vi "UTIL Config Analog Output_v3.vi"(0 "physical channels":tag) -> (1 "sampling info":cluster{"Fs":dbl, "#s":dbl}, 2 "error out":errorcluster, 3 "task out":refnum<k21>)   [LabVIEW 2010]
uses:
  <vilib>/DAQmx/create/channels.llb/DAQmx Create Channel (AO-Voltage-Basic).vi
  <vilib>/DAQmx/configure/timing.llb/DAQmx Timing (Sample Clock).vi
  Program Files (x86)/National Instruments/LabVIEW 2010/resource/objmgr/daqmx.rc
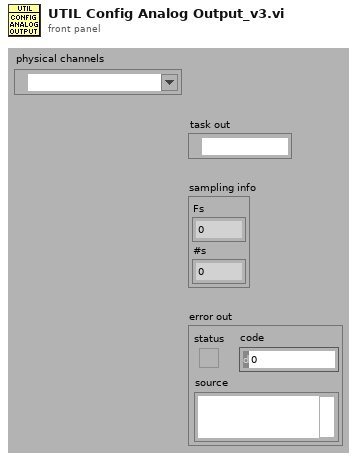
[diagram p1: front panel]
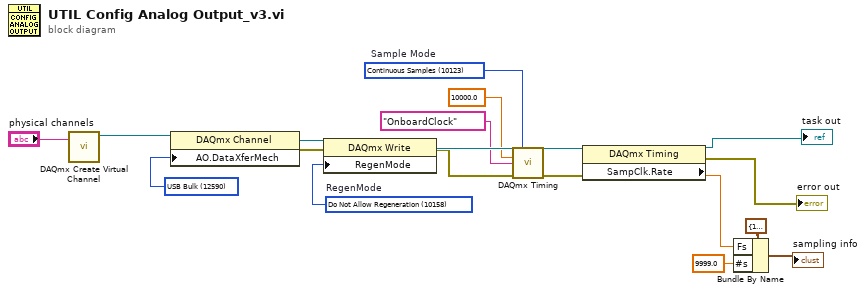
[diagram p0: block diagram]
diagram:
  w5 = 12590 items=["DMA"=10054, "Interrupts"=10204, "Programmed I/O"=10264, "USB Bulk"=12590] ("AO.DataXferMech")
  w10 = 10158 items=["Allow Regeneration"=10097, "Do Not Allow Regeneration"=10158]  # RegenMode
  w8 = 10123 items=["Finite Samples"=10178, "Continuous Samples"=10123, "Hardware Timed Single Point"=12522]  # Sample Mode
  n1 = call-poly <vilib>:"DAQmx Create Virtual Channel.vi"("physical channels"="physical channels") -> ("task out"=w1:refnum<k21>)  [unwired: 13 in, 1 out]
  n2 = property class="DAQmx Channel"(reference=w1, "AO.DataXferMech"=w5) -> (reference out=w7:refnum<k21>, error out=w6:errorcluster)  [unwired: 1 in]
  n3 = property class="DAQmx Write"(reference=w7, error in=w6, "RegenMode"=w10) -> (reference out=w14:refnum<k21>, error out=w9:errorcluster)
  n4 = call-poly <vilib>:"DAQmx Timing.vi"("task/channels in"=w14, "sample mode"=w8, "rate"=10000.0, "source"=tag "OnboardClock" ("Sample Clock Source"), "error in"=w9) -> ("task out"=w12:refnum<k21>, "error out"=w13:errorcluster)  [unwired: 9 in]
  n5 = property class="DAQmx Timing"(reference=w12, error in=w13) -> (reference out=→"task out":refnum<k21>, error out=→"error out":errorcluster, "SampClk.Rate"=w18:dbl)
  n6 = Bundle By Name(cluster=cluster{"Fs":dbl, "#s":dbl} {"Fs"=1000.0, "#s"=1000.0} ("sampling info"), "Fs"=w18, "#s"=9999.0) -> (→"sampling info":cluster{"Fs":dbl, "#s":dbl})
